vi "Voltage - HW-Timed Single Point Output.vi"() -> ()   [LabVIEW 2022 SP3]
doc: "This example demonstrates how to continuously generate analog output data using hardware timed, single point writes. This means that for each loop iteration, the VI writes a single sample to device. The device will then output that sample on the next tick of the sample clock. If an additional sample clock tick occurs before the next data point is written to the device, an error will be thrown indicating that this has happened. To ignore these errors, set the \"Convert Late Errors To Warnings\" control to TRUE.\n\nHardware Timed Single Point output works best when using a deterministic operating system (such as LabVIEW Real-Time). Because of the less deterministic nature of general purpose operating systems (such as Microsoft Windows), the software loop will not always take the exact same amount of time to execute, and this may lead to the occasional missed sample clock. If missed sample clock errors become an issue, you can try decreasing the sample rate, or setting the \"Convert Late Errors To Warnings\" control to TRUE.\n\nRefer to your device documentation for pinouts and hardware capabilities."
uses:
  <vilib>/Utility/error.llb/DialogType.ctl
  <vilib>/DAQmx/write.llb/DAQmx Write (Analog 1D DBL NChan 1Samp).vi
  <vilib>/DAQmx/create/channels.llb/DAQmx Create Channel (AO-Voltage-Basic).vi
  <vilib>/DAQmx/configure/timing.llb/DAQmx Timing (Sample Clock).vi
  <vilib>/DAQmx/miscellaneous.llb/DAQmx Fill In Error Info.vi
  <resource>/objmgr/daqmx.rc
  <vilib>/ptbypt/NI_PtbyPt.lvlib
panel:
  in  "Convert Late Errors to Warnings":bool
  in  "Output Array":T1(array[cluster])=[{"Waveform Type"=enum."Sine Wave", "Amplitude"=1.0, "Frequency"=10.0}] {"Frequency" format="%0.2p"; "Amplitude" format="%0.2p"}
  in  "Stop":bool
  in  "Sample Rate":dbl=100.0
  in  "Sample Clock Source":tag="OnboardClock"
  in  "Max Voltage":dbl=5.0
  in  "Min Voltage":dbl=-5.0
  in  "Physical Channel(s)":tag="Dev1/ao0"
  out "Actual Sample Rate":dbl=100.0 format="%0.2f"
  out "Waveform Chart":dbl[][](graph)
  # "Channel Settings"
  # "Output"
  # "Waveform Settings"
  # "Timing and Buffer Settings"
  # "The number of elements in the waveform array must equal the number of channels in the task."
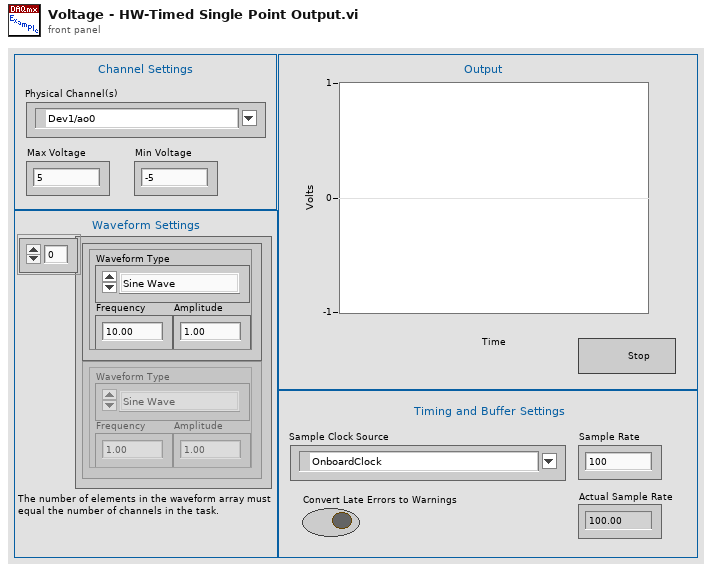
[diagram p1: front panel]
types:
  T1 = cluster{"Waveform Type":enum16{"Sine Wave", "Triangle Wave", "Square Wave", "Sawtooth Wave"}, "Amplitude":dbl, "Frequency":dbl}[]
  T2 = typedef "DialogType.ctl" = u16
  T3 = enum16{"Sine Wave", "Triangle Wave", "Square Wave", "Sawtooth Wave"}
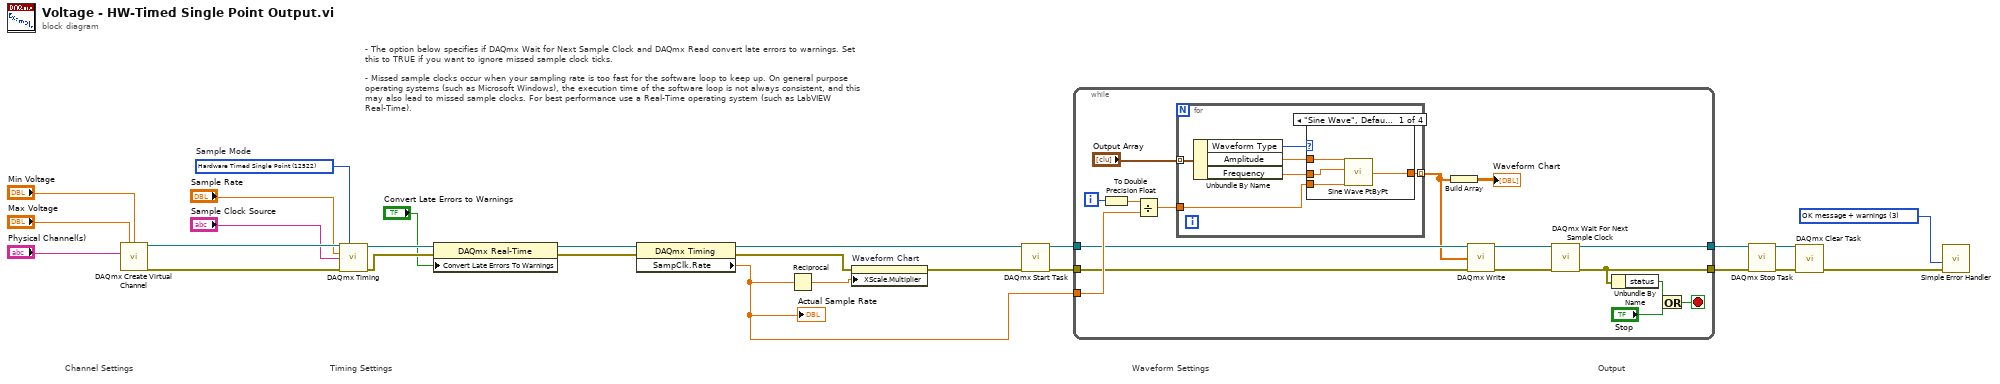
[diagram p0: block diagram]
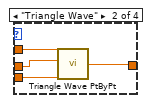
[diagram p2: hidden frame]
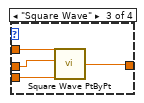
[diagram p3: hidden frame]
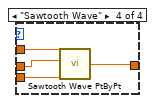
[diagram p4: hidden frame]
diagram:
  w3 = T2 3 items=["no dialog", "OK message", "continue or stop message", "OK message + warnings", "continue/stop + warnings"] ("type of dialog (OK msg:1)")
  w26 = 12522 items=["Finite Samples"=10178, "Continuous Samples"=10123, "Hardware Timed Single Point"=12522]  # Sample Mode
  # "- The option below specifies if DAQmx Wait for Next Sample Clock and DAQmx Read convert late errors to warnings. Set this to TRUE if you want to ignore missed sample clock ticks.\n \n- Missed sample clocks occur when your sampling rate is too fast for the software loop to keep up. On general purpose operating systems (such as Microsoft Windows), the execution time of the software loop is not always consistent, and this may also lead to missed sample clocks. For best performance use a Real-Time operating system (such as LabVIEW Real-Time)."
  # "Output"
  # "Waveform Settings"
  # "Timing Settings"
  # "Channel Settings"
  n1 = call-poly <vilib>:"DAQmx Create Virtual Channel.vi"("maximum value"="Max Voltage", "minimum value"="Min Voltage", "physical channels"="Physical Channel(s)") -> ("task out"=w24:refnum<k21>, "error out"=w25:errorcluster)  [unwired: 11 in]
  n2 = call-poly <vilib>:"DAQmx Timing.vi"("task/channels in"=w24, "sample mode"=w26, "rate"="Sample Rate", "source"="Sample Clock Source", "error in"=w25) -> ("task out"=w9:refnum<k21>, "error out"=w8:errorcluster)  [unwired: 9 in]
  n3 = property class="DAQmx Real-Time"(reference=w9, error in=w8, "Convert Late Errors To Warnings"="Convert Late Errors to Warnings") -> (reference out=w11:refnum<k21>, error out=w10:errorcluster)
  n4 = property class="DAQmx Timing"(reference=w11, error in=w10) -> (reference out=w2:refnum<k21>, error out=w5:errorcluster, "SampClk.Rate"=w4:dbl)
  "Actual Sample Rate" <- w4
  n5 = Reciprocal(x=w4) -> (1/x=w6:dbl)
  n6 = property on="Waveform Chart" class="WFChart (strict)"(error in=w5, "XScale.Multiplier"=w6) -> (error out=w1:errorcluster)  [unwired: 1 in, 1 out]
  n7 = call <vilib>:"DAQmx Start Task.vi"("task/channels in"=w2, "error in"=w1) -> ("task out"=w23:refnum<k21>, "error out"=w22:errorcluster)  [unwired: 12 in]
  n8 = while {
    tunnel: w23 -> [w30]
    tunnel: w22 -> [w29]
    tunnel: [w33] -> w12
    tunnel: [w34] -> w13
    tunnel: w4 -> [w38]
    i -> [w37]
    stop <- w42 stop-if-true
    n9 = To Double Precision Float(number=w37) -> (double precision float=w36:dbl)
    n10 = Divide(x=w36, y=w38) -> (x/y=w35:dbl)
    n11 = for {
      tunnel: "Output Array" -> [w48] mode=indexing
      tunnel: w35 -> [w44]
      tunnel: [w43] -> w28 mode=indexing
      n12 = Unbundle By Name(w48) -> ("Waveform Type"=w47:T3, "Amplitude"=w46:dbl, "Frequency"=w45:dbl)
      n13 = case shown="\"Sine Wave\", Default" w47 {
        tunnel: w46 -> [w52 w54 w58 w64]
        tunnel: w45 -> [w51 w55 w59 w62]
        tunnel: w44 -> [w50 w56 w60 w63]
        tunnel: [w49 w53 w57 w61] -> w43
        frame "Sine Wave", Default {
          n14 = call <vilib>:"Sine Wave PtByPt.vi"("time"=w50, "frequency"=w51, "amplitude"=w52) -> ("sine wave"=w49:dbl)  [unwired: 1 in]
        }
        frame "Triangle Wave" {
          n15 = call <vilib>:"Triangle Wave PtByPt.vi"("time"=w56, "frequency"=w55, "amplitude"=w54) -> ("triangle wave"=w53:dbl)  [unwired: 1 in]
        }
        frame "Square Wave" {
          n16 = call <vilib>:"Square Wave PtByPt.vi"("amplitude"=w58, "frequency"=w59, "time"=w60) -> ("square wave"=w57:dbl)  [unwired: 2 in]
        }
        frame "Sawtooth Wave" {
          n17 = call <vilib>:"Sawtooth Wave PtByPt.vi"("time"=w63, "frequency"=w62, "amplitude"=w64) -> ("sawtooth wave"=w61:dbl)  [unwired: 1 in]
        }
      }
    }
    n18 = Build Array(w28) -> (→"Waveform Chart":dbl[][])
    n19 = call-poly <vilib>:"DAQmx Write.vi"("task/channels in"=w30, "data"=w28, "error in"=w29) -> ("task out"=w32:refnum<k21>, "error out"=w31:errorcluster)  [unwired: 10 in, 1 out]
    n20 = call <vilib>:"DAQmx Wait For Next Sample Clock.vi"("task/channels in"=w32, "error in"=w31) -> ("task out"=w34:refnum<k21>, "error out"=w33:errorcluster)  [unwired: 11 in, 1 out]
    n21 = Unbundle By Name(w33) -> ("status"=w41:bool)
    n22 = Or(x=w41, y="Stop") -> (x .or. y?=w42:bool)
  }
  n23 = call <vilib>:"DAQmx Stop Task.vi"("task/channels in"=w13, "error in"=w12) -> ("task out"=w15:refnum<k21>, "error out"=w14:errorcluster)  [unwired: 12 in]
  n24 = call <vilib>:"DAQmx Clear Task.vi"("task in"=w15, "error in"=w14) -> ("error out"=w21:errorcluster)  [unwired: 13 in]
  n25 = call <vilib>:"Simple Error Handler.vi"("type of dialog (OK msg:1)"=w3, "error in (no error)"=w21) -> ()  [unwired: 3 in, 5 out]
